vi "shortcutMenuSelected.vi"(8 "error in (no error)":errorcluster, 10 "matlabScript":string, 11 "ExperimentRunner in":refnum<class "ExperimentRunner.lvclass">) -> (0 "error out":errorcluster, 3 "ExperimentRunner out":refnum<class "ExperimentRunner.lvclass">)   [LabVIEW 2011, in "Views.lvlib" / "ExperimentControl.lvlib" / "ExperimentRunner.lvclass"]
uses:
  ExperimentRunner.lvclass
  MatlabScripts/MatlabScripts.lvclass
  ExperimentRunner.lvclass/ExperimentRunner.ctl
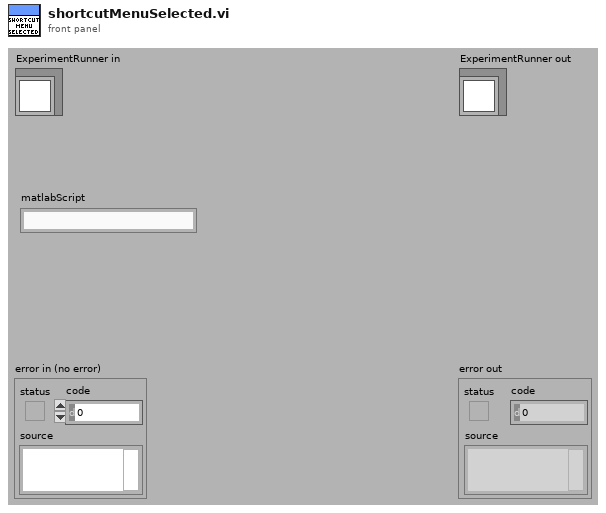
[diagram p1: front panel]
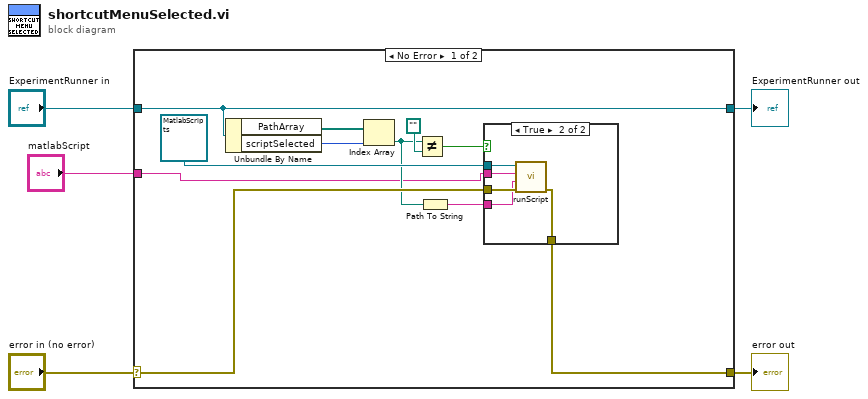
[diagram p0: block diagram]
diagram:
  n1 = case shown="No Error" "error in (no error)" {
    selector: "error in (no error)" -> [w15 w24]
    tunnel: [w14 w24] -> w4
    tunnel: [w13 w23] -> w2
    tunnel: "ExperimentRunner in" -> [w13 w23]
    tunnel: "matlabScript" -> [w6 _]
    frame No Error {
      n2 = Unbundle By Name(w13) -> ("PathArray"=w12:path[], "scriptSelected"=w11:i32)
      n3 = Index Array(array=w12, index=w11) -> (element=w8:path)
      n4 = Not Equal?(x=w8, y=path "") -> (x != y?=w9:bool)
      n5 = Path To String(path=w8) -> (string=w7:string)
      n6 = case shown="True" w9 {
        tunnel: refnum<class "MatlabScripts.lvclass"> refnum ("Views.lvlib:ExperimentControl.lvlib:MatlabScripts.lvclass") -> [_ w22]
        tunnel: w6 -> [_ w21]
        tunnel: w15 -> [w17 w20]
        tunnel: [w17 w19] -> w14
        tunnel: w7 -> [_ w18]
        frame False {
        }
        frame True {
          n7 = call "runScript.vi"("error in (no error)"=w20, "script"=w18, "matlabScript"=w21, "MatlabScripts in"=w22) -> ("error out"=w19:errorcluster)  [unwired: 6 in, 1 out]
        }
      }
    }
    frame Error {
    }
  }
  "error out" <- w4
  "ExperimentRunner out" <- w2
